vi "client.vi"(0 "Network Manager IP Address or Hostname":string, 1 "Network Manager port":u16=1875, 2 "timeout ms":i32=10000, 3 "Service name":string, 4 "function name":string, 5 "error in":errorcluster, 6 "args":variant, 7 "kwargs":variant, 8 "username":string, 9 "password":string) -> (14 "result":variant, 19 "error out":errorcluster)   [LabVIEW 2010]
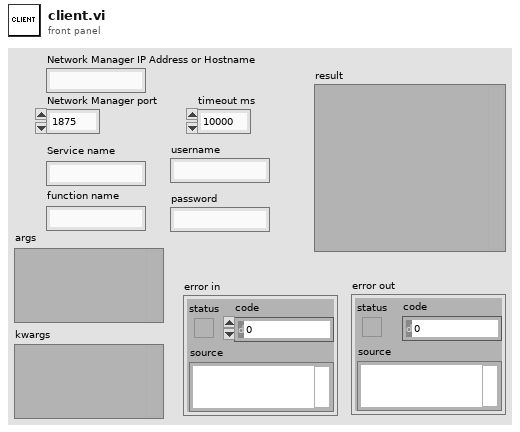
[diagram p1: front panel]
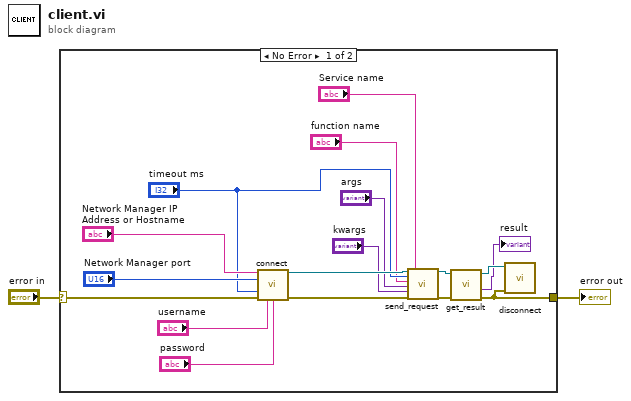
[diagram p0: block diagram]
diagram:
  n1 = case shown="No Error" "error in" {
    selector: "error in" -> [w5 w20]
    tunnel: [w6 w20] -> w2
    frame No Error {
      n2 = call "connect.vi"("Network Manager IP Address or Hostname"="Network Manager IP Address or Hostname", "Network Manager port"="Network Manager port", "timeout ms"="timeout ms", "error in"=w5, "username"="username", "password"="password") -> ("connection ID"=w17:refnum<k5>, "error out"=w15:errorcluster)  [unwired: 7 in, 1 out]
      n3 = call "send_request.vi"("connection ID"=w17, "timeout ms"="timeout ms", "function name"="function name", "args"="args", "kwargs"="kwargs", "error in"=w15, "Service name"="Service name") -> ("connection ID out"=w13:refnum<k5>, "error out"=w11:errorcluster)  [unwired: 9 in, 2 out]
      n4 = call "get_result.vi"("error in"=w11, "connection ID"=w13) -> ("error out"=w6:errorcluster, "result"=→"result":variant, "connection ID out"=w10:refnum<k5>)  [unwired: 6 in, 1 out]
      n5 = call "disconnect.vi"("error in (no error)"=w6, "connection ID"=w10) -> ()  [unwired: 9 in, 1 out]
    }
    frame Error {
    }
  }
  "error out" <- w2
